vi "R45.vi"() -> ()   [LabVIEW 2016, in "Beamline Sections.lvlib"]
uses:
  Beamline Sections.lvlib
  <vilib>/Instr/_visa.llb/VISA Open Access Mode.ctl
  main/save load/saveload.ctl
panel:
  out "error out 3":errorcluster
  out "error out 4":errorcluster
  out "error out":errorcluster
  out "read current quad B 2":string
  out "error out 2":errorcluster
  out "r45 end x steerer read":dbl
  in  "Tab Control":enum32{"Control", "Readbacks"}(tab)
  in  "gfm setAmps":dbl(knob) min=0.0 max=150.0 scale=0.0..100.0
  in  "ExB #2 Electric":dbl(knob) min=0.0 max=200.0 scale=0.0..40.0
  in  "Reset ExB 2":bool
  in  "ExB #1 Electric":dbl(knob) min=0.0 max=200.0 scale=0.0..46.0
  out "Trans Steerer Y Read":dbl format="%#.2g"
  out "Trans Steerer X Read":dbl format="%#.2g"
  in  "R45 Y steerer":dbl(knob) min=-10.0 max=10.0 scale=-10.0..8.0
  in  "R45 Quad A":dbl(knob) min=0.0 max=200.0 scale=10.0..120.0
  in  "R45 X steerer":dbl(knob) min=-10.0 max=10.0 scale=-10.0..10.0
  out "Transmission\n Steerer range":bool
  out "R45 quad Range":bool
  in  "R45 Quad B":dbl(knob) min=0.0 max=200.0 scale=50.0..80.0
  in  "stop":bool
  out "ExB":bool
  out "ExB Voltage Read-":dbl format="%#.2g"
  in  "ExB#1 Magnet":dbl
  in  "Cluster":T1
  out "ExB Voltage Read +":dbl format="%#.2g"
  out "read current quad a":string
  out "read voltage quad A":string
  out "read current quad B":string
  out "read voltage Quad B":string
  in  "R45 X steerer end":dbl(knob) min=-10.0 max=10.0 scale=-10.0..10.0
  in  "ExB#2 Magnet":dbl
  out "gfm read":string
  out "ExB#1 +READ I":dbl
  out "ExB - I":dbl
  out "R45 steer +X I":dbl
  out "R45 steer -X  I":dbl
  out "R45 steer +Y I":dbl
  out "R45 steer -Y I":dbl
  out "R45 steer +X":dbl
  out "R45 steer -X":dbl
  out "R45 steer +Y":dbl
  out "R45 steer -Y":dbl
  out "R45 steer +X Set":dbl
  out "R45 steer -X Set":dbl
  out "R45 steer +Y Set":dbl
  out "R45 steer -Y Set":dbl
  out "Switch magnet field readback":dbl=0.8365 min=0.0 max=1.6
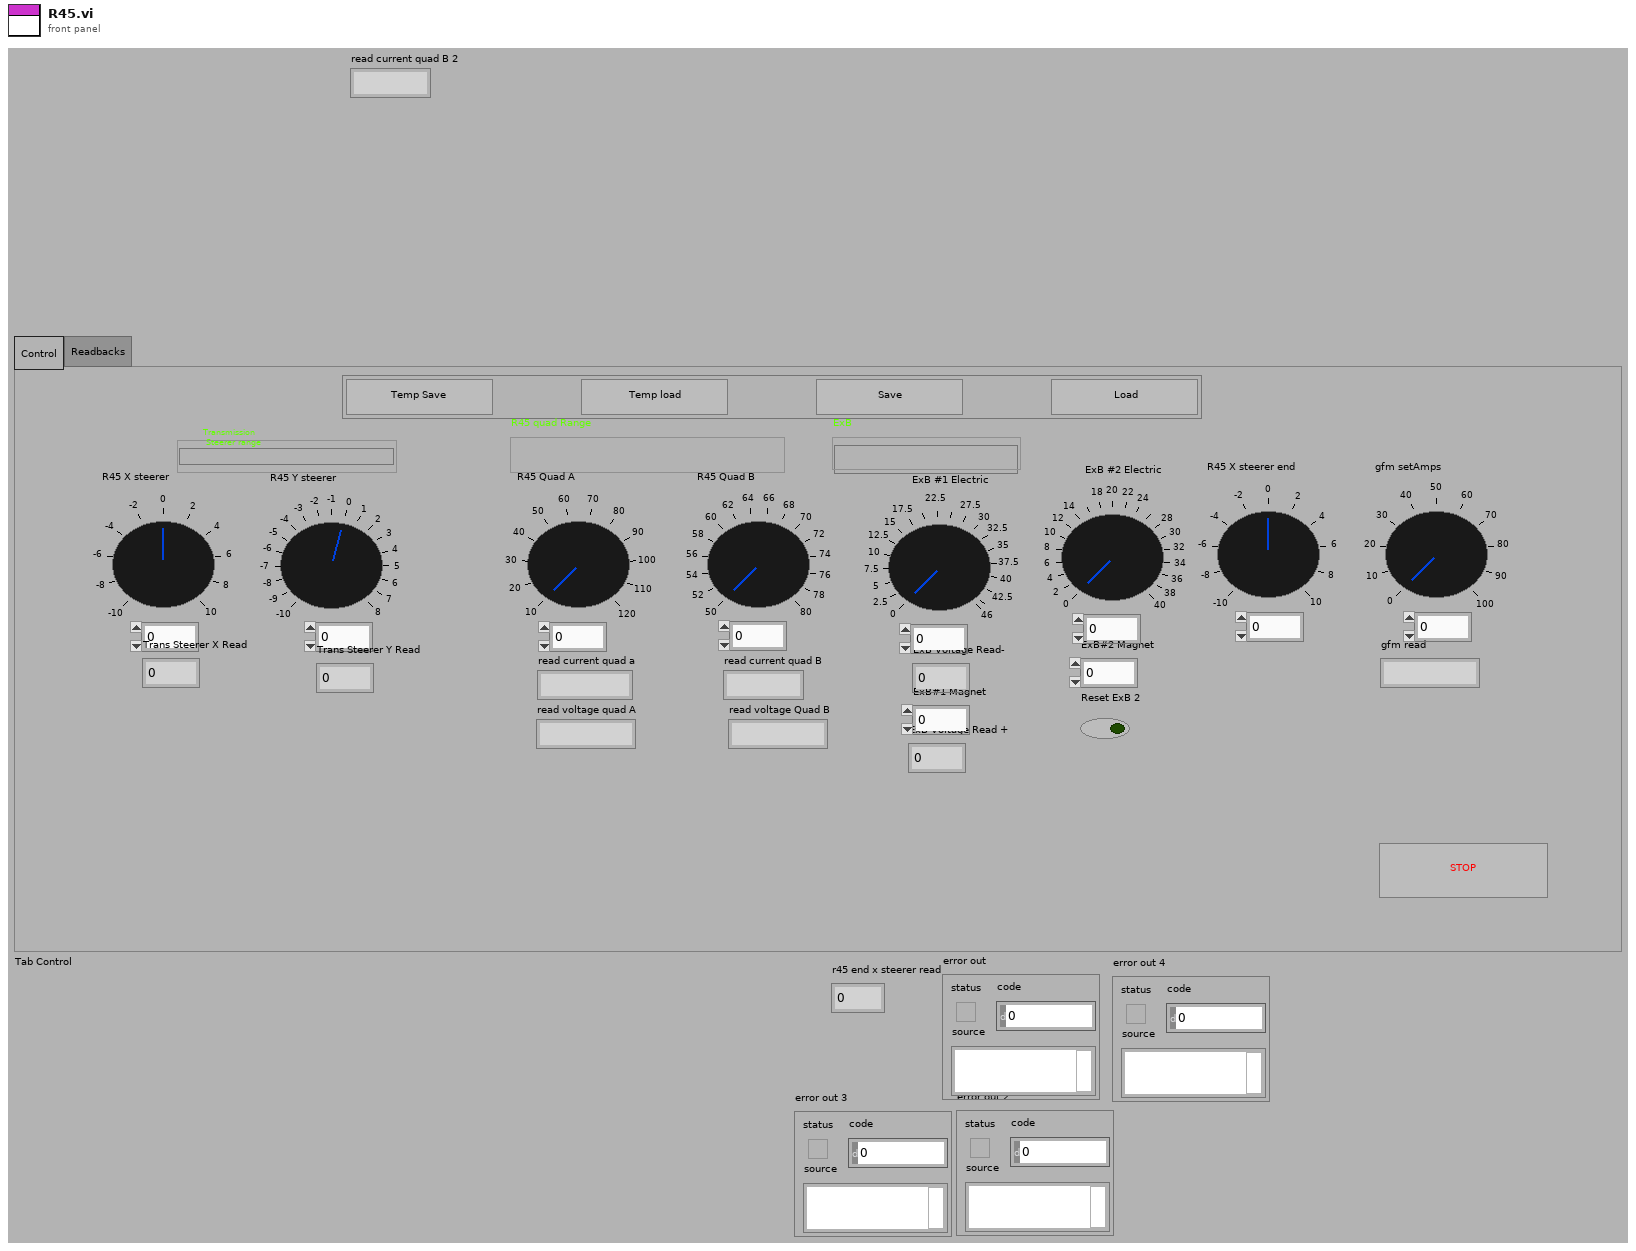
[diagram p1: front panel]
types:
  T1 = typedef "main.lvlib/saveload.ctl" = cluster{"OK Button":bool, "OK Button 2":bool, "OK Button 3":bool, "OK Button 4":bool}
  T2 = typedef "VISA Open Access Mode.ctl" = u32
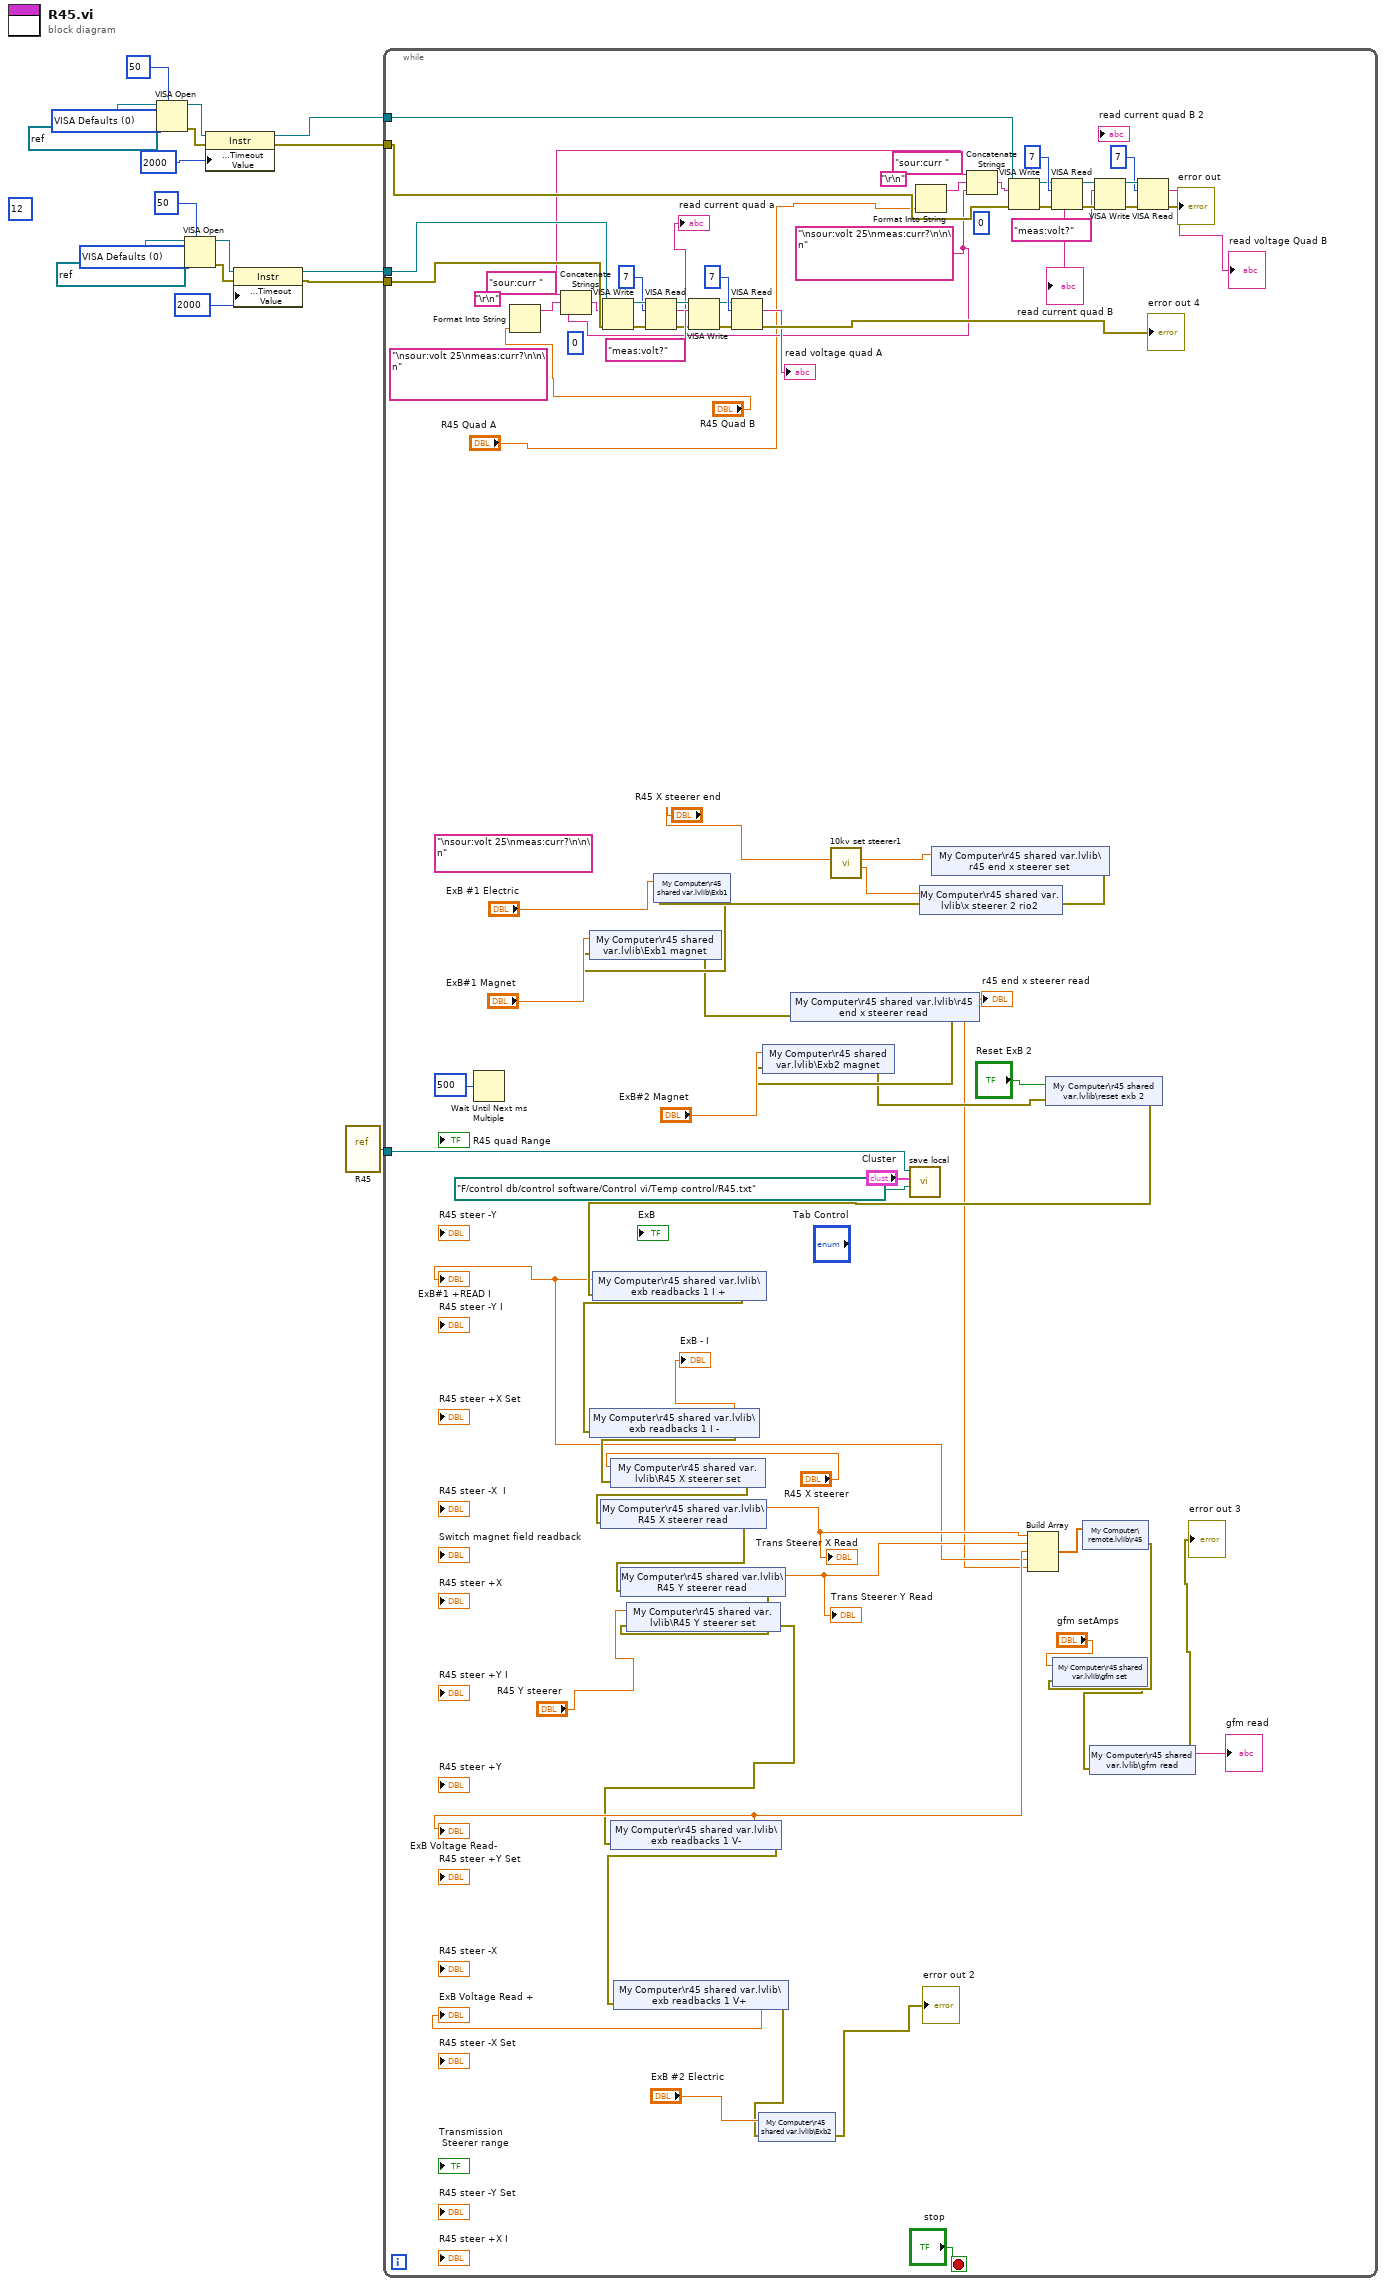
[diagram p0: block diagram]
diagram:
  w15 = T2 0 items=["VISA Defaults"=0, "Exclusive Lock"=1, "Load Configured Settings"=4] ("Access Mode")
  w5 = T2 0 items=["VISA Defaults"=0, "Exclusive Lock"=1, "Load Configured Settings"=4] ("Access Mode")
  (unwired) u16 12 ("Device\nAddress(1)")
  n1 = VISA Open(timeout (0)=u32 50 ("VISA Open timeout (0)"), access mode=w15, VISA resource name=refnum<visa-resource-name> "GPIB1::3::INSTR" ("VISA GPIB Resource")) -> (VISA resource name=w12:refnum<visa-resource-name>, error out=w11:errorcluster)  [unwired: 2 in]
  n2 = VISA Open(timeout (0)=u32 50 ("VISA Open timeout (0)"), access mode=w5, VISA resource name=refnum<visa-resource-name> "GPIB1::6::INSTR" ("VISA GPIB Resource")) -> (VISA resource name=w9:refnum<visa-resource-name>, error out=w10:errorcluster)  [unwired: 2 in]
  n3 = property class="Instr"(reference=w12, error in=w11, "General Settings:Timeout Value"=u32 2000) -> (reference out=w4:refnum<visa-resource-name>, error out=w1:errorcluster)
  n4 = property class="Instr"(reference=w9, error in=w10, "General Settings:Timeout Value"=u32 2000) -> (reference out=w3:refnum<visa-resource-name>, error out=w2:errorcluster)
  n5 = vi-ref "R45.vi"() -> (w17:refnum<vi>)
  n6 = while {
    tunnel: w17 -> [w96]
    tunnel: w4 -> [w52]
    tunnel: w3 -> [w50]
    tunnel: w2 -> [w51]
    tunnel: w1 -> [w45]
    stop <- "stop" stop-if-true
    (unwired) "\r\n"
    (unwired) i16 0 ("mode (0)")
    w42 = "sour:curr " ("string")
    w43 = "\nsour:volt 25\nmeas:curr?\n\n\n" ("write buffer")
    (unwired) "\r\n"
    (unwired) i16 0 ("mode (0)")
    (unwired) "sour:curr " ("string")
    (unwired) "\nsour:volt 25\nmeas:curr?\n\n\n" ("write buffer")
    (unwired) "\nsour:volt 25\nmeas:curr?\n\n\n" ("write buffer")
    n7 = Wait Until Next ms Multiple(millisecond multiple=u32 500) -> ()  [unwired: 1 out]
    n8 = Format Into String("R45 Quad B") -> (resulting string=w53:string)  [unwired: 3 in, 1 out]
    n9 = Concatenate Strings(w42, w53, w43) -> (w40:string)
    n10 = VISA Write(VISA resource name=w50, write buffer=w40, error in (no error)=w51) -> (VISA resource name out=w56:refnum<visa-resource-name>, error out=w55:errorcluster)  [unwired: 1 out]
    n11 = VISA Read(VISA resource name=w56, byte count=u32 7, error in (no error)=w55) -> (VISA resource name out=w59:refnum<visa-resource-name>, read buffer=→"read current quad a":string, error out=w60:errorcluster)  [unwired: 1 out]
    n12 = VISA Write(VISA resource name=w59, write buffer="meas:volt?", error in (no error)=w60) -> (VISA resource name out=w57:refnum<visa-resource-name>, error out=w62:errorcluster)  [unwired: 1 out]
    n13 = VISA Read(VISA resource name=w57, byte count=u32 7, error in (no error)=w62) -> (read buffer=→"read voltage quad A":string, error out=→"error out 4":errorcluster)  [unwired: 2 out]
    n14 = call "10kv set steerer1.vi"("Steerer Control IN"="R45 X steerer end") -> ("- Steerer"=w21:dbl, "+ Steerer"=w20:dbl)  [unwired: 8 in, 1 out]
    n15 = call "save local.vi"("file path (use dialog)"=path "F:/control db/control software/Control vi/Temp control/R45.txt", "Ring"="Cluster", "VI Refnum"=w96) -> ()  [unwired: 2 out]
    n16 = Format Into String("R45 Quad A") -> (resulting string=w72:string)  [unwired: 3 in, 1 out]
    n17 = shared-variable "My Computer\\r45 shared var.lvlib\\x steerer 2 rio2"(w21) -> ()  [unwired: 1 in, 1 out]
    n18 = shared-variable "My Computer\\r45 shared var.lvlib\\r45 end x steerer set"(w20) -> (error out=w83:errorcluster)  [unwired: 1 in]
    n19 = shared-variable "My Computer\\r45 shared var.lvlib\\Exb1"("ExB #1 Electric", error in=w83) -> (error out=w82:errorcluster)
    n20 = shared-variable "My Computer\\r45 shared var.lvlib\\Exb1 magnet"("ExB#1 Magnet", error in=w82) -> (error out=w81:errorcluster)
    n21 = shared-variable "My Computer\\r45 shared var.lvlib\\r45 end x steerer read"(error in=w81) -> (w31:dbl, error out=w80:errorcluster)
    "r45 end x steerer read" <- w31
    n22 = shared-variable "My Computer\\r45 shared var.lvlib\\Exb2 magnet"("ExB#2 Magnet", error in=w80) -> (error out=w78:errorcluster)
    n23 = Concatenate Strings(w42, w72, w43) -> (w41:string)
    n24 = VISA Write(VISA resource name=w52, write buffer=w41, error in (no error)=w45) -> (VISA resource name out=w69:refnum<visa-resource-name>, error out=w70:errorcluster)  [unwired: 1 out]
    n25 = shared-variable "My Computer\\r45 shared var.lvlib\\reset exb 2"("Reset ExB 2", error in=w78) -> (error out=w77:errorcluster)
    n26 = shared-variable "My Computer\\r45 shared var.lvlib\\exb readbacks 1 I +"(error in=w77) -> (w32:dbl, error out=w39:errorcluster)
    "ExB#1 +READ I" <- w32
    n27 = shared-variable "My Computer\\r45 shared var.lvlib\\exb readbacks 1 I -"(error in=w39) -> (→"ExB - I":dbl, error out=w38:errorcluster)
    n28 = shared-variable "My Computer\\r45 shared var.lvlib\\R45 X steerer set"("R45 X steerer", error in=w38) -> (error out=w37:errorcluster)
    n29 = shared-variable "My Computer\\r45 shared var.lvlib\\R45 X steerer read"(error in=w37) -> (w35:dbl, error out=w36:errorcluster)
    "Trans Steerer X Read" <- w35
    n30 = shared-variable "My Computer\\r45 shared var.lvlib\\R45 Y steerer read"(error in=w36) -> (w34:dbl, error out=w85:errorcluster)
    "Trans Steerer Y Read" <- w34
    n31 = shared-variable "My Computer\\r45 shared var.lvlib\\R45 Y steerer set"("R45 Y steerer", error in=w85) -> (error out=w19:errorcluster)
    n32 = shared-variable "My Computer\\r45 shared var.lvlib\\exb readbacks 1 V-"(error in=w19) -> (w33:dbl, error out=w84:errorcluster)
    "ExB Voltage Read-" <- w33
    n33 = shared-variable "My Computer\\r45 shared var.lvlib\\exb readbacks 1 V+"(error in=w84) -> (→"ExB Voltage Read +":dbl, error out=w75:errorcluster)
    n34 = shared-variable "My Computer\\r45 shared var.lvlib\\Exb2"("ExB #2 Electric", error in=w75) -> (error out=→"error out 2":errorcluster)
    n35 = Build Array(w35, w34, w33, w32, w31) -> (w30:dbl[])
    n36 = VISA Read(VISA resource name=w69, byte count=u32 7, error in (no error)=w70) -> (VISA resource name out=w66:refnum<visa-resource-name>, read buffer=→"read current quad B":string, error out=w65:errorcluster)  [unwired: 1 out]
    n37 = shared-variable "My Computer\\remote.lvlib\\r45"(w30) -> (error out=w28:errorcluster)  [unwired: 1 in]
    n38 = shared-variable "My Computer\\r45 shared var.lvlib\\gfm set"("gfm setAmps", error in=w28) -> (error out=w27:errorcluster)
    n39 = shared-variable "My Computer\\r45 shared var.lvlib\\gfm read"(error in=w27) -> (→"gfm read":string, error out=→"error out 3":errorcluster)
    n40 = VISA Write(VISA resource name=w66, write buffer="meas:volt?", error in (no error)=w65) -> (VISA resource name out=w68:refnum<visa-resource-name>, error out=w63:errorcluster)  [unwired: 1 out]
    n41 = VISA Read(VISA resource name=w68, byte count=u32 7, error in (no error)=w63) -> (read buffer=→"read voltage Quad B":string, error out=→"error out":errorcluster)  [unwired: 2 out]
  }
